vi "JAUS Header Decoder.vi"(4 "Encoded JAUS Message":string) -> (8 "Jaus Version [0]":u8, 10 "Message Type (0-5)":u8, 12 "HC flags (6-7)":u8, 14 "Data Size (8-23)":u16, 16 "HC Number (24-31)":u8, 18 "HC Length (32-39)":u8, 20 "Priority(40-41)":u8, 21 "Broadcast Flags (42-43)":u8, 22 "Ack/Nak (44-45)":u8, 23 "Data Flags (46-47)":u8, 24 "Destination ID (48-79)":u32, 25 "Source ID (80-95)":u32, 26 "Payload":string, 27 "Sequence Number (16 bits)":u16)   [LabVIEW 2011]
uses:
  Address.ctl
panel:
  out "Destination":T1={"Subsystem Id"=90, "Node Id"=1, "Component Id"=1}
  out "Source":T1={"Subsystem Id"=90, "Node Id"=1, "Component Id"=1}
  out "Message size":i32
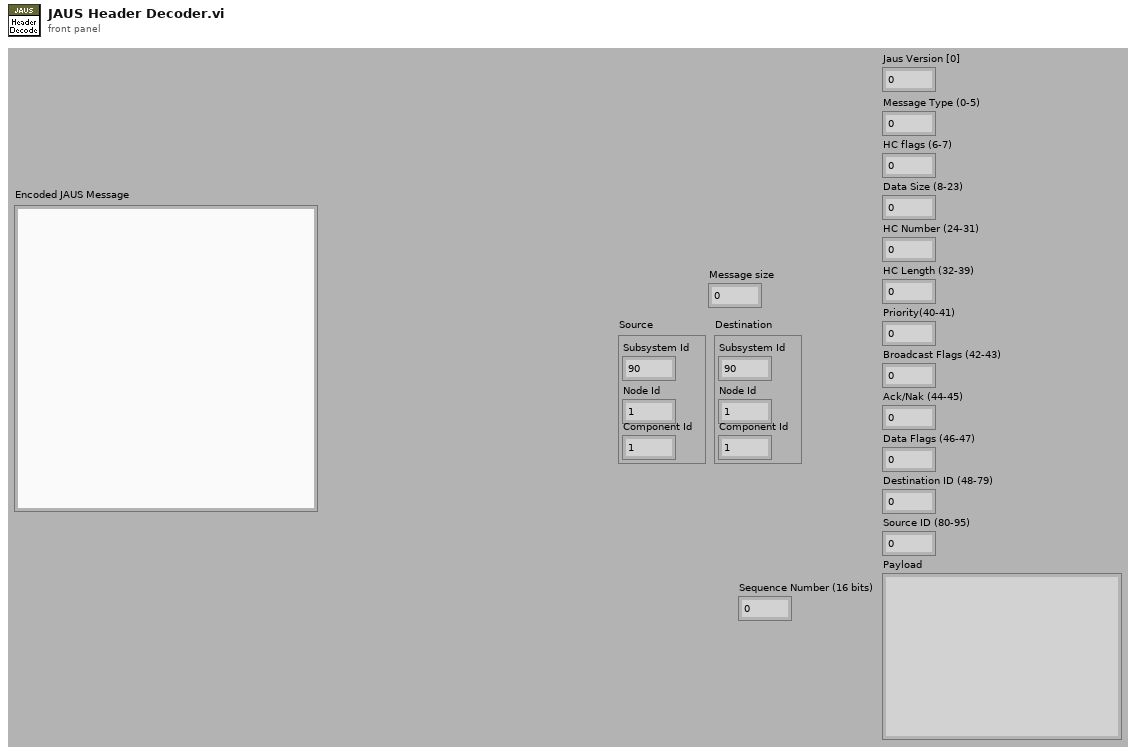
[diagram p1: front panel]
types:
  T1 = typedef "Address.ctl" = cluster{"Subsystem Id":u16, "Node Id":u8, "Component Id":u8}
  T2 = cluster{"Boolean array[0]":bool, "Boolean array[1]":bool, "Boolean array[2]":bool, "Boolean array[3]":bool, "Boolean array[4]":bool, "Boolean array[5]":bool, "Boolean array[6]":bool, "Boolean array[7]":bool}
  T3 = cluster{"[0]":u8, "[1]":u8, "[2]":u8, "[3]":u8, "[4]":u8, "[5]":u8, "[6]":u8, "[7]":u8, "[8]":u8, "[9]":u8, "[10]":u8, "[11]":u8, "[12]":u8, "[13]":u8, "[14]":u8}
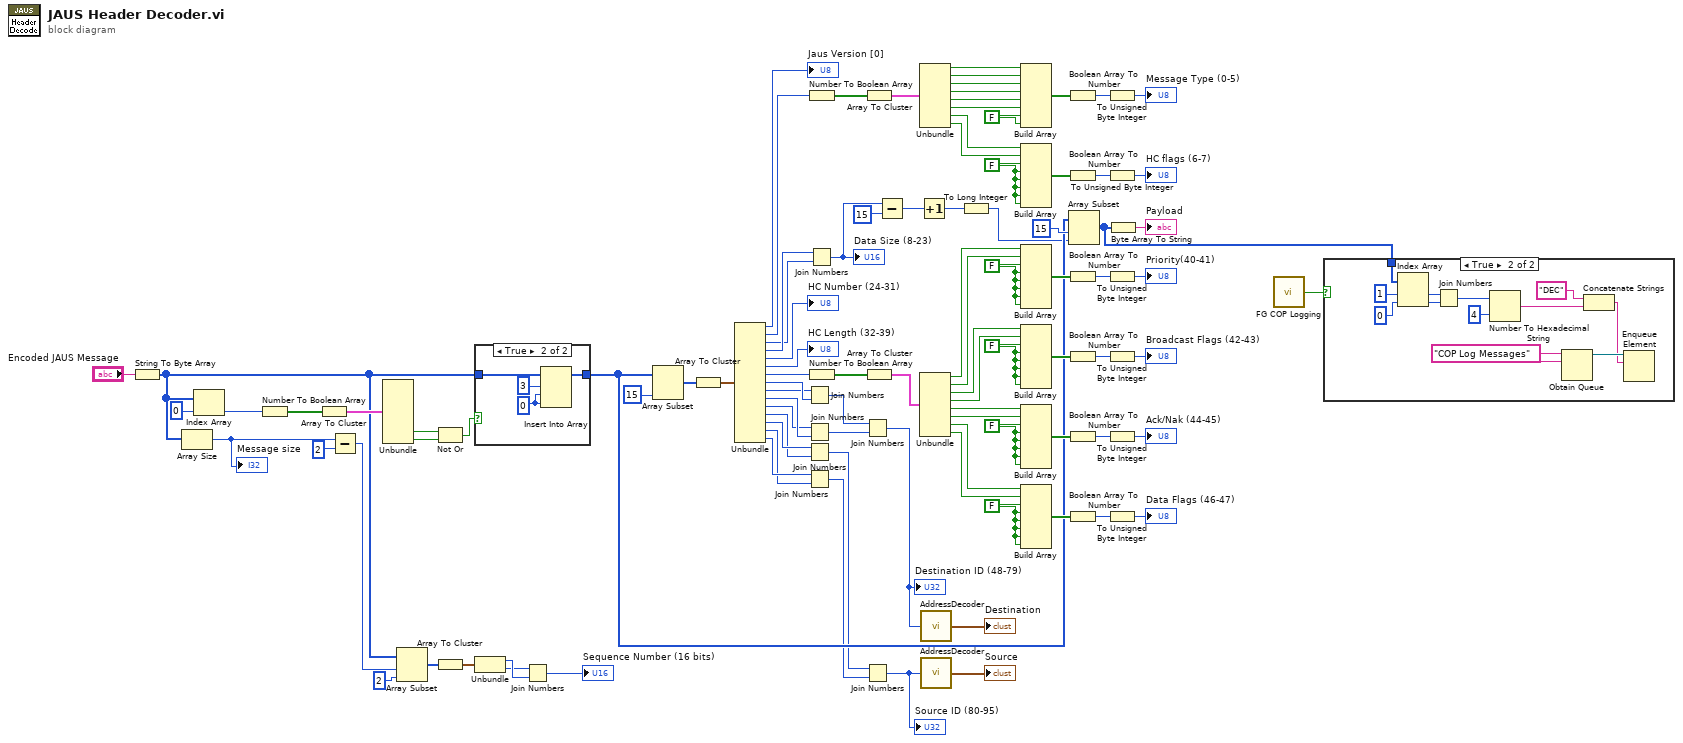
[diagram p0: block diagram]
diagram:
  w53 = FALSE ("element")
  w52 = FALSE ("element")
  w51 = FALSE ("element")
  w50 = FALSE ("element")
  w73 = FALSE ("element")
  w79 = FALSE ("element")
  n1 = String To Byte Array(string="Encoded JAUS Message") -> (unsigned byte array=w4:u8[])
  n2 = Array Size(array=w4) -> (size(s)=w7:i32)
  "Message size" <- w7
  n3 = Index Array(array=w4, index=0) -> (element=w44:u8)
  n4 = Number To Boolean Array(number=w44) -> (Boolean array=w35:bool[])
  n5 = Array To Cluster(array=w35) -> (cluster=w45:T2)
  n6 = Subtract(x=w7, y=2) -> (x-y=w6:i32)
  n7 = Unbundle(w45) -> ("Boolean array[6]"=w43:bool, "Boolean array[7]"=w42:bool)  [unwired: 6 out]
  n8 = Array Subset(array=w4, index=w6, length=2) -> (w93:u8[])
  n9 = Not Or(1:w42, 2:w43) -> (0:w41:bool)
  n10 = Array To Cluster(array=w93) -> (cluster=w94:cluster{"[0]":u8, "[1]":u8})
  n11 = case shown="True" w41 {
    tunnel: w4 -> [w99 w103]
    tunnel: [w99 w102] -> w40
    frame False {
    }
    frame True {
      w100 = u8 0 ("new element/subarray")
      n12 = Insert Into Array(array=w103, index=3, new element #1=w100, new element #2=w100) -> (w102:u8[])
    }
  }
  n13 = Unbundle(w94) -> ("[0]"=w39:u8, "[1]"=w38:u8)
  n14 = Join Numbers(hi=w38, lo=w39) -> ((hi.lo)=→"Sequence Number (16 bits)":u16)
  n15 = Array Subset(array=w40, length=15) -> (w37:u8[])  [unwired: 1 in]
  n16 = Array To Cluster(array=w37) -> (cluster=w97:T3)
  n17 = Unbundle(w97) -> ("[0]"=→"Jaus Version [0]":u8, "[1]"=w34:u8, "[2]"=w23:u8, "[3]"=w24:u8, "[4]"=→"HC Number (24-31)":u8, "[5]"=→"HC Length (32-39)":u8, "[6]"=w30:u8, "[7]"=w29:u8, "[8]"=w28:u8, "[9]"=w27:u8, "[10]"=w26:u8, "[11]"=w17:u8, "[12]"=w18:u8, "[13]"=w16:u8, "[14]"=w25:u8)
  n18 = Join Numbers(hi=w28, lo=w29) -> ((hi.lo)=w22:u16)
  n19 = Join Numbers(hi=w26, lo=w27) -> ((hi.lo)=w21:u16)
  n20 = Join Numbers(hi=w18, lo=w17) -> ((hi.lo)=w20:u16)
  n21 = Join Numbers(hi=w25, lo=w16) -> ((hi.lo)=w19:u16)
  n22 = Number To Boolean Array(number=w34) -> (Boolean array=w86:bool[])
  n23 = Join Numbers(hi=w24, lo=w23) -> ((hi.lo)=w9:u16)
  "Data Size (8-23)" <- w9
  n24 = Number To Boolean Array(number=w30) -> (Boolean array=w71:bool[])
  n25 = Join Numbers(hi=w22, lo=w21) -> ((hi.lo)=w13:u32)
  "Destination ID (48-79)" <- w13
  n26 = Join Numbers(hi=w20, lo=w19) -> ((hi.lo)=w15:u32)
  "Source ID (80-95)" <- w15
  n27 = Array To Cluster(array=w86) -> (cluster=w85:T2)
  n28 = Array To Cluster(array=w71) -> (cluster=w72:T2)
  n29 = Subtract(x=w9, y=u16 15) -> (x-y=w8:u16)
  n30 = Increment(x=w8) -> (x+1=w10:u16)
  n31 = Unbundle(w85) -> ("Boolean array[0]"=w81:bool, "Boolean array[1]"=w80:bool, "Boolean array[2]"=w82:bool, "Boolean array[3]"=w83:bool, "Boolean array[4]"=w84:bool, "Boolean array[5]"=w76:bool, "Boolean array[6]"=w75:bool, "Boolean array[7]"=w74:bool)
  n32 = Unbundle(w72) -> ("Boolean array[0]"=w61:bool, "Boolean array[1]"=w60:bool, "Boolean array[2]"=w59:bool, "Boolean array[3]"=w58:bool, "Boolean array[4]"=w57:bool, "Boolean array[5]"=w56:bool, "Boolean array[6]"=w55:bool, "Boolean array[7]"=w54:bool)
  n33 = call "AddressDecoder.vi"("Address"=w13) -> ("Address Cluster"=→"Destination":T1)
  n34 = call "AddressDecoder.vi"("Address"=w15) -> ("Address Cluster"=→"Source":T1)
  n35 = To Long Integer(number=w10) -> (32bit integer=w2:i32)
  n36 = Build Array(w81, w80, w82, w83, w84, w76, w79, w79) -> (w78:bool[])
  n37 = Build Array(w75, w74, w73, w73, w73, w73, w73, w73) -> (w77:bool[])
  n38 = Build Array(w61, w60, w50, w50, w50, w50, w50, w50) -> (w70:bool[])
  n39 = Build Array(w59, w58, w51, w51, w51, w51, w51, w51) -> (w49:bool[])
  n40 = Build Array(w57, w56, w52, w52, w52, w52, w52, w52) -> (w48:bool[])
  n41 = Build Array(w55, w54, w53, w53, w53, w53, w53, w53) -> (w47:bool[])
  n42 = Boolean Array To Number(Boolean array=w78) -> (number=w89:u32)
  n43 = Boolean Array To Number(Boolean array=w77) -> (number=w90:u32)
  n44 = Boolean Array To Number(Boolean array=w70) -> (number=w69:u32)
  n45 = Boolean Array To Number(Boolean array=w49) -> (number=w68:u32)
  n46 = Boolean Array To Number(Boolean array=w48) -> (number=w67:u32)
  n47 = Boolean Array To Number(Boolean array=w47) -> (number=w66:u32)
  n48 = Array Subset(array=w40, index=15, length=w2) -> (w1:u8[])
  n49 = To Unsigned Byte Integer(number=w89) -> (unsigned 8bit integer=→"Message Type (0-5)":u8)
  n50 = To Unsigned Byte Integer(number=w90) -> (unsigned 8bit integer=→"HC flags (6-7)":u8)
  n51 = To Unsigned Byte Integer(number=w69) -> (unsigned 8bit integer=→"Priority(40-41)":u8)
  n52 = To Unsigned Byte Integer(number=w68) -> (unsigned 8bit integer=→"Broadcast Flags (42-43)":u8)
  n53 = To Unsigned Byte Integer(number=w67) -> (unsigned 8bit integer=→"Ack/Nak (44-45)":u8)
  n54 = To Unsigned Byte Integer(number=w66) -> (unsigned 8bit integer=→"Data Flags (46-47)":u8)
  n55 = Byte Array To String(unsigned byte array=w1) -> (string=→"Payload":string)
  n56 = call "FG COP Logging.vi"() -> ("Logging? out"=w3:bool)  [unwired: 2 in]
  n57 = case shown="True" w3 {
    tunnel: w1 -> [_ w115]
    frame False {
    }
    frame True {
      w108 = "COP Log Messages" ("name (unnamed)")
      n58 = Index Array(array=w115, index #1=1 ("index"), index #2=0 ("index")) -> (element #1=w111:u8, element #2=w112:u8)
      n59 = Join Numbers(hi=w111, lo=w112) -> ((hi.lo)=w109:u16)
      n60 = Number To Hexadecimal String(1:i16 4 ("width (-)"), 2:w109) -> (0:w107:string)
      n61 = Obtain Queue(name (unnamed)=w108, element data type=w108) -> (queue out=w106:refnum<queue>)  [unwired: 3 in, 2 out]
      n62 = Concatenate Strings("DEC" ("string"), w107) -> (w105:string)
      n63 = Enqueue Element(queue=w106, element=w105) -> ()  [unwired: 2 in, 3 out]
    }
  }
